vi "Calculate Transparency Mask.vi"(11 "Picture in":picture) -> (2 "mask":u8[](array[numeric]), 3 "24-bit pixmap":u32[][](array[numeric]), 5 "top left":cluster{"x":i16, "y":i16})   [LabVIEW 2020, in "PieChart.lvclass"]
uses:
  PieChart.lvclass
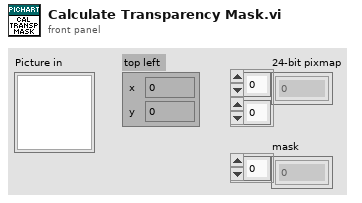
[diagram p1: front panel]
types:
  T1 = typedef "imagedata.ctl" = cluster{"image type":i32, "image depth":i32, "image":u8[], "mask":u8[], "colors":u32[], "Rectangle":cluster{"left":i16, "top":i16, "right":i16, "bottom":i16}}
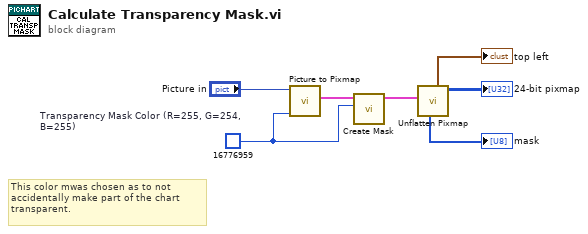
[diagram p0: block diagram]
diagram:
  w7 = u32 16776959  # Transparency Mask Color (R=255, G=254, B=255)
  # "This color mwas chosen as to not \naccidentally make part of the chart\ntransparent."
  n1 = call <vilib>:"Picture to Pixmap.vi"("Background Color"=w7, "picture"="Picture in") -> ("image data"=w5:T1)  [unwired: 8 in, 1 out]
  n2 = call <vilib>:"Create Mask.vi"("Mask Color (Black)"=w7, "image data"=w5) -> ("image data"=w6:T1)  [unwired: 9 in]
  n3 = call <vilib>:"Unflatten Pixmap.vi"("image data"=w6) -> ("24-bit pixmap"=→"24-bit pixmap":u32[][], "top left"=→"top left":cluster{"x":i16, "y":i16}, "mask"=→"mask":u8[])  [unwired: 4 in, 4 out]
